vi "Read Sequence Call Step Dictionary.vi"(8 "error in (no error)":errorcluster, 11 "Measurement Interface in":refnum<class "Measurement Interface.lvclass">) -> (0 "error out":errorcluster, 2 "Sequence Call Step Dictionary.lvlibp:Sequence Call Step Dict":refnum<class "Sequence Call Step Dictionary.lvclass">, 3 "Measurement Interface out":refnum<class "Measurement Interface.lvclass">)   [LabVIEW 2016, in "Measurement Interface.lvlib" / "Measurement Interface.lvclass"]
uses:
  Measurement Interface.lvclass
  Plugins/Sequence Call Step Dictionary.lvlibp/Sequence Call Step Dictionary.lvclass
  Measurement Interface.lvclass/Measurement Interface.ctl
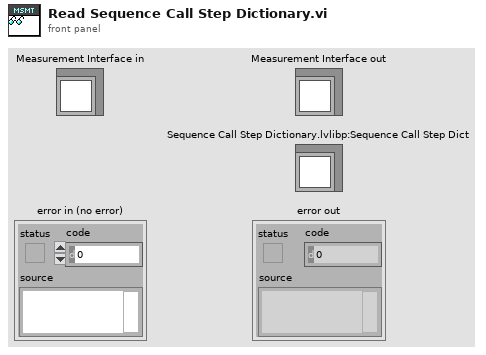
[diagram p1: front panel]
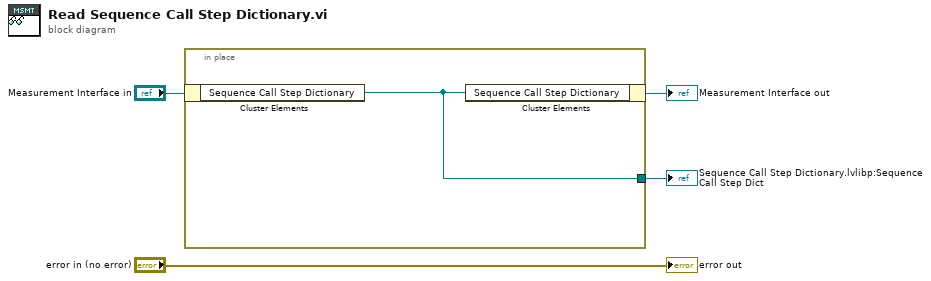
[diagram p0: block diagram]
diagram:
  n1 = in-place {
    in-place-border: [w5] -> w1
    n2 = in-place-cluster #1("Measurement Interface in") -> ("Sequence Call Step Dictionary"=w5:refnum<class "Sequence Call Step Dictionary.lvclass">)
    n3 = in-place-cluster #1("Sequence Call Step Dictionary"=w5) -> (→"Measurement Interface out":refnum<class "Measurement Interface.lvclass">)
  }
  "Sequence Call Step Dictionary.lvlibp:Sequence Call Step Dict" <- w1
  "error out" <- "error in (no error)"
